vi "Tabulate_Plotted_data.vi"(3 "Data":string[][](array[string]), 4 "Channel Names":string[](array[string]), 5 "Channels to Tabulate":i32[](listbox)) -> (0 "spreadsheet string":string, 1 "Channel Values":string[][](array[string]), 2 "Channel Names":string[](array[string]))   [LabVIEW 2020]
uses:
  Results_plotter_Global.vi
  Data plotting/subVIs/Plot_Values_Global.vi
panel:
  out "Table":string[][](table)
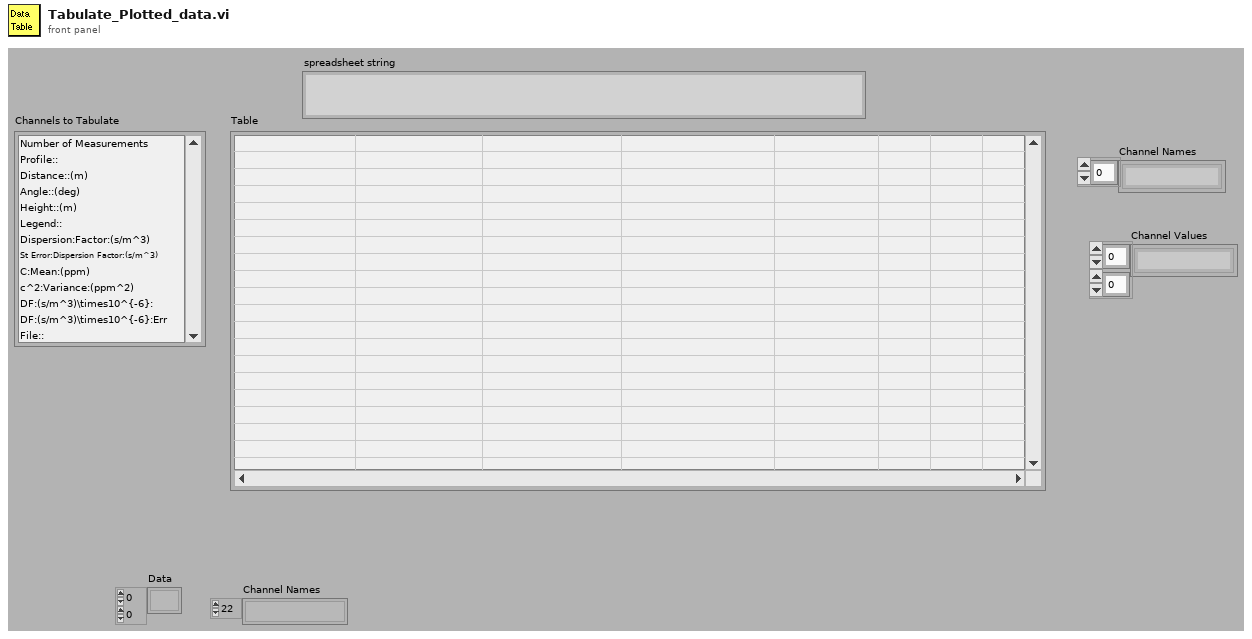
[diagram p1: front panel]
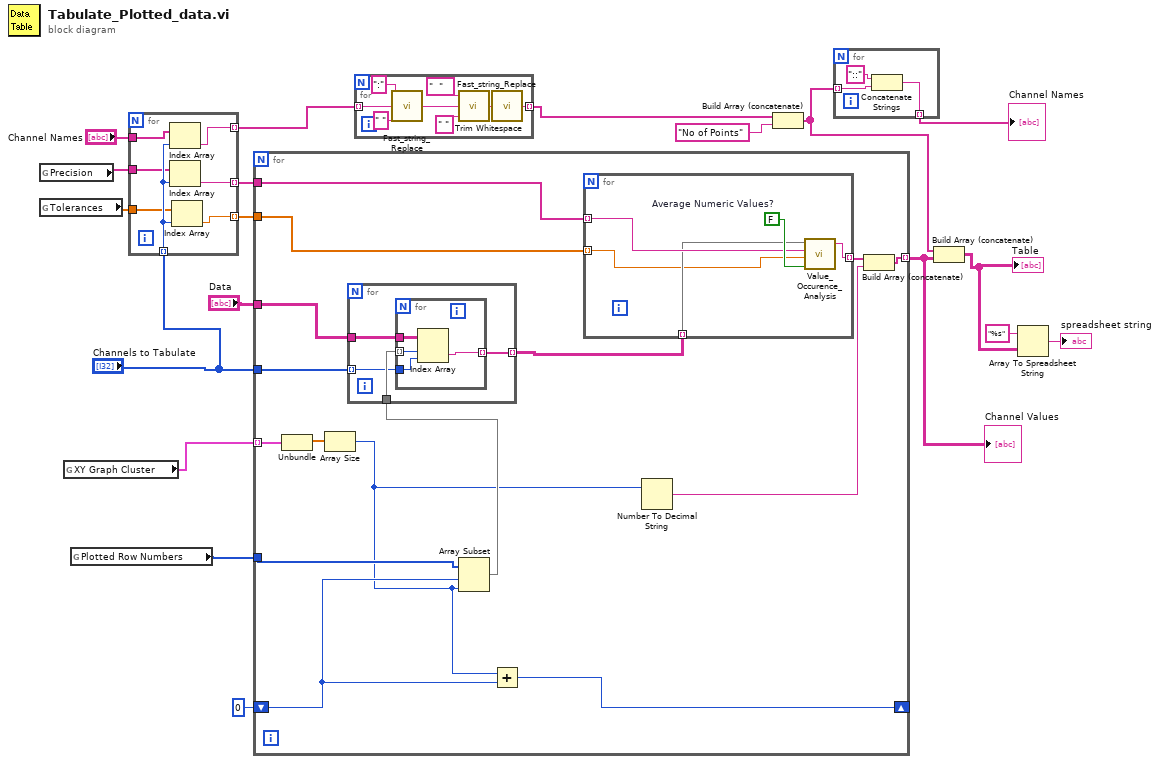
[diagram p0: block diagram]
diagram:
  n1 = global read "Results_plotter_Global.vi" "Precision"() -> (w16:string[])
  n2 = global read "Results_plotter_Global.vi" "Tolerances"() -> (w15:dbl[])
  n3 = global read "Plot_Values_Global.vi" "XY Graph Cluster"() -> (w1:cluster{dbl[], dbl[]}[])
  n4 = global read "Results_plotter_Global.vi" "Plotted Row Numbers"() -> (w2:i32[])
  n5 = for {
    tunnel: "Channels to Tabulate" -> [w26] mode=indexing
    tunnel: "Channel Names" -> [w25]
    tunnel: w16 -> [w24]
    tunnel: w15 -> [w23]
    tunnel: [w22] -> w14 mode=indexing
    tunnel: [w21] -> w13 mode=indexing
    tunnel: [w20] -> w6 mode=indexing
    n6 = Index Array(array=w25, index=w26) -> (element=w20:string)
    n7 = Index Array(array=w24, index=w26) -> (element=w22:string)
    n8 = Index Array(array=w23, index=w26) -> (element=w21:dbl)
  }
  n9 = for {
    tunnel: w1 -> [w40] mode=indexing
    shift-right: [w37] -> _
    shift-left: 0 -> [w38]
    tunnel: w2 -> [w39]
    tunnel: "Data" -> [w35]
    tunnel: "Channels to Tabulate" -> [w34]
    tunnel: w14 -> [w33]
    tunnel: w13 -> [w32]
    tunnel: [w29] -> w12 mode=indexing
    n10 = Unbundle(w40) -> (w41:dbl[])  [unwired: 1 out]
    n11 = Array Size(array=w41) -> (size(s)=w28:i32)
    n12 = Array Subset(array=w39, index=w38, length=w28) -> (w36:i32[])
    n13 = for {
      tunnel: w36 -> [w45]
      tunnel: w35 -> [w44]
      tunnel: w34 -> [w43] mode=indexing
      tunnel: [w42] -> w31 mode=indexing
      n14 = for {
        tunnel: w45 -> [w49] mode=indexing
        tunnel: w44 -> [w48]
        tunnel: w43 -> [w47]
        tunnel: [w46] -> w42 mode=indexing
        n15 = Index Array(array=w48, index (row)=w49, index (col)=w47) -> (element=w46:string)
      }
    }
    n16 = Add(x=w28, y=w38) -> (x+y=w37:i32)
    n17 = for {
      tunnel: w33 -> [w53] mode=indexing
      tunnel: w32 -> [w50] mode=indexing
      tunnel: [w52] -> w30 mode=indexing
      tunnel: w31 -> [w51] mode=indexing
      w54 = FALSE  # Average Numeric Values?
      n18 = call "Value_Occurence_Analysis.vi"("Average Numeric Values?"=w54, "Tolerance"=w50, "Precision (3)"=w53, "String Array"=w51) -> ("Output String"=w52:string)  [unwired: 2 out]
    }
    n19 = Number To Decimal String(number=w28) -> (decimal integer string=w27:string)  [unwired: 1 out]
    n20 = Build Array (concatenate)(w30, w27) -> (w29:string[])
  }
  "Channel Values" <- w12
  n21 = for {
    tunnel: w6 -> [w62] mode=indexing
    tunnel: [w59] -> w5 mode=indexing
    n22 = call "Fast_string_Replace.vi"("Replace match with:"=" ", "Input String"=w62, "regular expression"=":") -> ("Output String"=w58:string)  [unwired: 2 out]
    n23 = call "Fast_string_Replace.vi"("Replace match with:"=" ", "Input String"=w58, "regular expression"="  ") -> ("Output String"=w57:string)  [unwired: 2 out]
    n24 = call <vilib>:"Trim Whitespace.vi"("string"=w57) -> ("trimmed string"=w59:string)  [unwired: 1 in]
  }
  n25 = Build Array (concatenate)(w5, "No of Points") -> (w3:string[])
  n26 = for {
    tunnel: w3 -> [w64] mode=indexing
    tunnel: [w63] -> w4 mode=indexing
    n27 = Concatenate Strings("::" ("regular expression"), w64) -> (w63:string)
  }
  "Channel Names" <- w4
  n28 = Build Array (concatenate)(w3, w12) -> (w10:string[][])
  "Table" <- w10
  n29 = Array To Spreadsheet String(array=w10, 3:"%s" ("format string")) -> (spreadsheet string=→"spreadsheet string":string)  [unwired: 1 out]
